vi "Print Error.vi"(7 "error out":errorcluster) -> ()   [LabVIEW 2009]
uses:
  Program Files/National Instruments/LabVIEW 2009/Targets/NI/RT/vi.lib/NI_Real-Time Target Support.lvlib
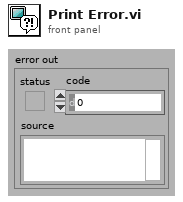
[diagram p1: front panel]
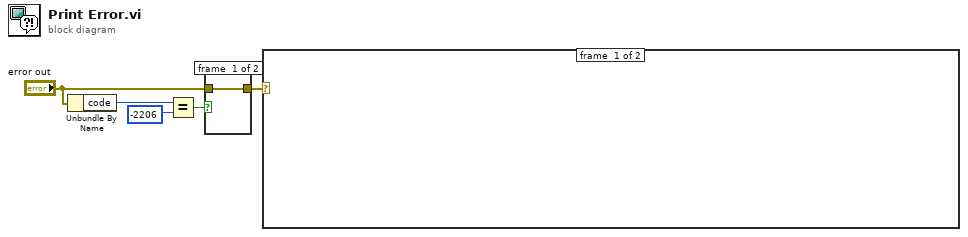
[diagram p0: block diagram]
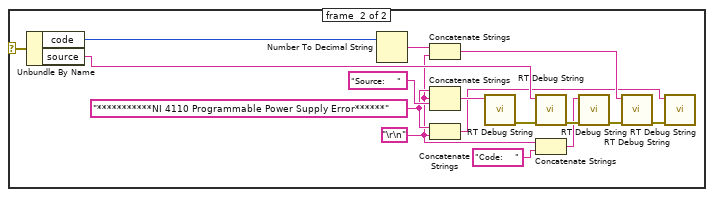
[diagram p3: hidden frame]
diagram:
  n1 = Unbundle By Name("error out") -> ("code"=w5:i32)
  n2 = Equal?(x=w5, y=-2206) -> (x = y?=w3:bool)
  n3 = case shown="True" w3 {
    tunnel: "error out" -> [w6 _]
    tunnel: [w6 _] -> w1
    frame #0 {
    }
    frame #1 {
    }
  }
  n4 = case shown="Error" w1 {
    selector: w1 -> [_ w20]
    frame #0 {
    }
    frame #1 {
      w8 = "\r\n"
      w9 = "***********NI 4110 Programmable Power Supply Error******" ("String")
      n5 = Unbundle By Name(w20) -> ("code"=w18:i32, "source"=w19:string)
      n6 = Number To Decimal String(number=w18) -> (decimal integer string=w13:string)  [unwired: 1 in]
      n7 = Concatenate Strings(w13, w8) -> (w12:string)
      n8 = Concatenate Strings(w9, w8, "Source:    " ("String")) -> (w22:string)
      n9 = Concatenate Strings(w9, w8) -> (w7:string)
      n10 = call "RT Debug String.vi"("String to write"=w22) -> ("error out"=w21:errorcluster)  [unwired: 10 in]
      n11 = call "RT Debug String.vi"("error in (no error)"=w21, "String to write"=w19) -> ("error out"=w17:errorcluster)  [unwired: 9 in]
      n12 = Concatenate Strings(w8, "Code:    " ("String")) -> (w14:string)
      n13 = call "RT Debug String.vi"("error in (no error)"=w17, "String to write"=w14) -> ("error out"=w11:errorcluster)  [unwired: 9 in]
      n14 = call "RT Debug String.vi"("error in (no error)"=w11, "String to write"=w12) -> ("error out"=w10:errorcluster)  [unwired: 9 in]
      n15 = call "RT Debug String.vi"("error in (no error)"=w10, "String to write"=w7) -> ()  [unwired: 9 in, 1 out]
    }
  }
